vi "Fetch Waveform.vi"(7 "Bind Source Channel (2: None)":i32(ring)=2 items=["Sub Source 0", "Sub Source 1", "None"], 8 "error in (no error)":errorcluster, 9 "Timeout (10000)":u32=10000, 10 "Source Channel (0: Channel 1)":i32(ring) items=["Channel 1"=0, "Channel 2"=1, "Channel 3"=2, "Channel 4"=3, "Waveform Memory 1"=5, "Waveform Memory 2"=6, "Serial Bus 1"=7, "Serial Bus 2"=8, "Digital Bus Low"=9, "Digital Bus High "=10, "Digital Bus 1"=11, "Digital Bus 2"=12, "External"=29, "Function 1"=32, "Function 2"=33, "Function 3"=34, "Function 4"=35, "Math 1"=36, "Math 2"=37, "Math 3"=38, "Math 4"=39, "FFT"=40, "Analog Bus"=41, "Pod 1"=42, "Pod 2"=43], 11 "VISA resource name":refnum<visa-resource-name>) -> (0 "error out":errorcluster, 2 "Waveform Data":waveform(dbl)(graph), 3 "VISA resource name out":refnum<visa-resource-name>)   [LabVIEW 2015, in "Agilent 2000 3000 X-Series.lvlib"]
doc: "Returns the waveform the oscilloscope acquired for the specified channel. The waveform is from an acquisition that you initiate prior to calling this VI.\n\nYou use the <b>Initiate</b> VI to start an acquisition on the channels that you enable with the <b>Configure Channel</b> VI. The oscilloscope acquires waveforms for the enabled channels concurrently. You must call this VI separately for each enabled channel to obtain the waveforms.\n\nYou can call the <b>Read Waveform</b> VI instead of using low-level VIs.\n\n<B>Note(s):</B>\nUse this VI only with other low-level VIs. The high-level VIs automatically incorporate this functionality. This VI does not check the instrument status."
uses:
  Agilent 2000 3000 X-Series.lvlib
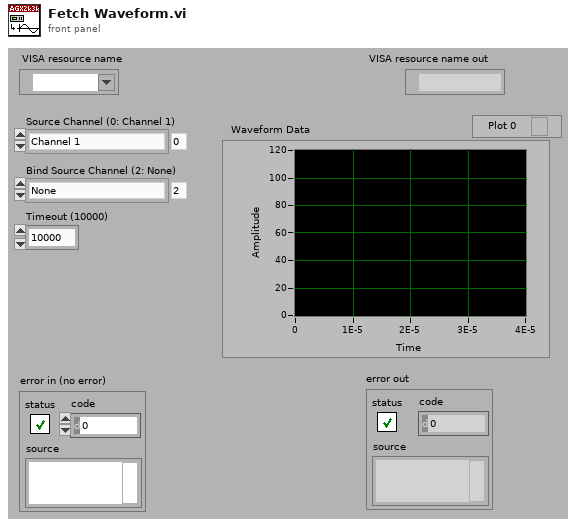
[diagram p1: front panel]
types:
  T1 = typedef "Agilent 2000 3000 X-Series.lvlib/Extended User Data.ctl" = cluster{"X-Series Mode":u16, "Acquisition Type (0: Normal)":i32}
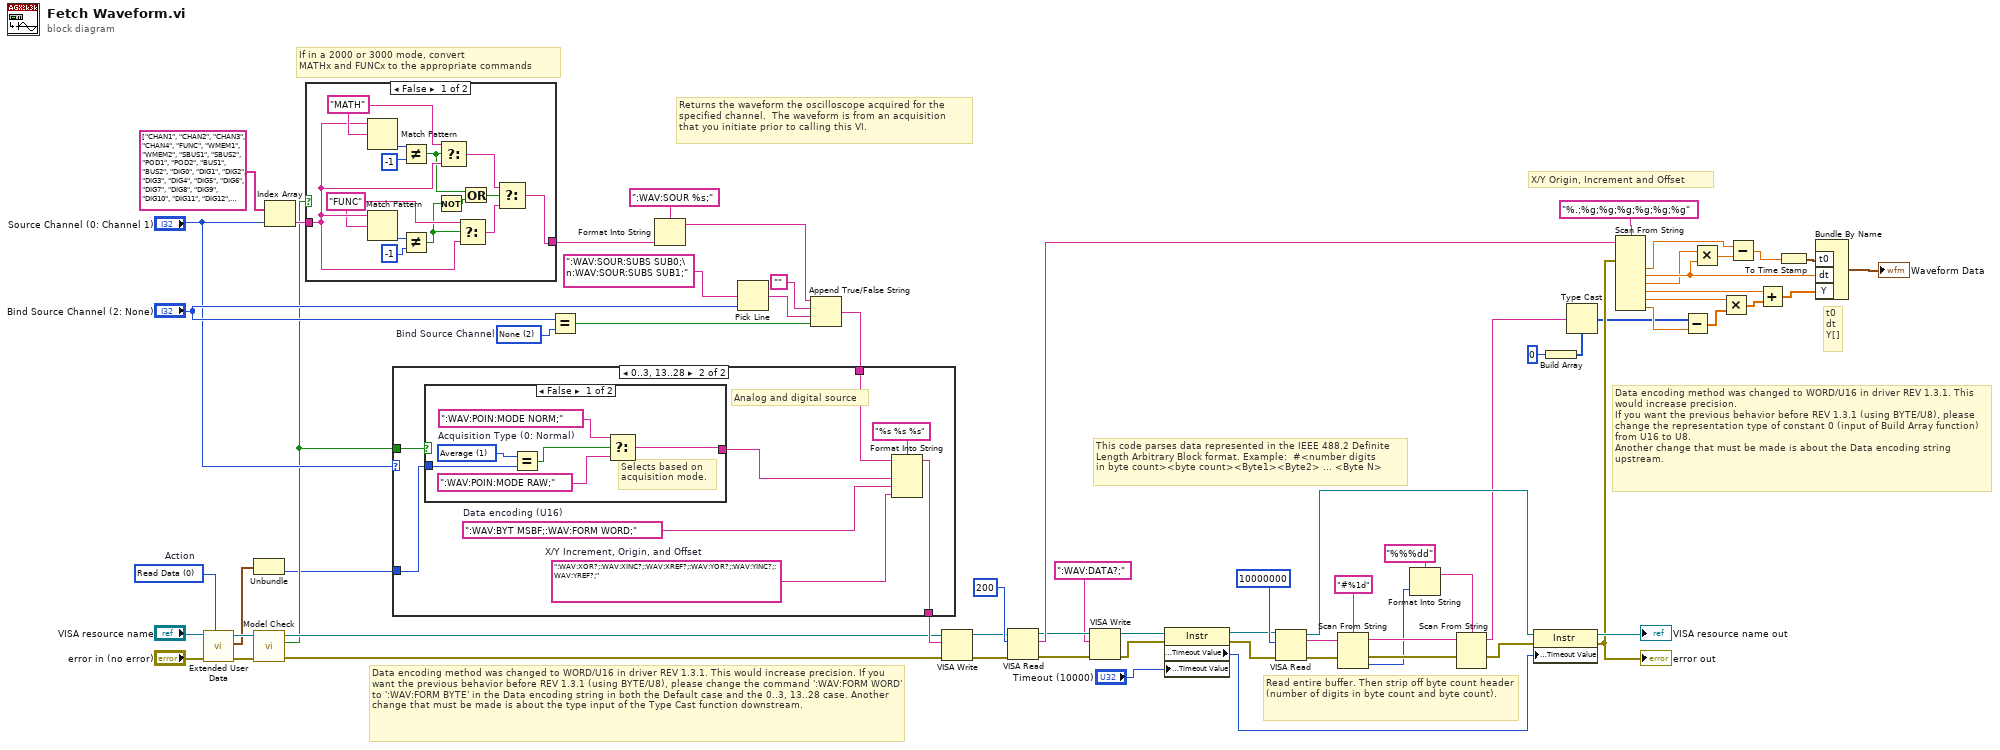
[diagram p0: block diagram]
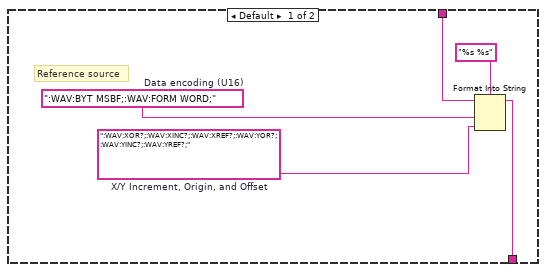
[diagram p3: hidden frame]
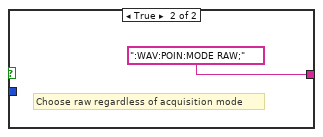
[diagram p4: hidden frame]
diagram:
  w4 = 0 items=["Read Data", "Write Data", "Clear Data", "Clear ALL Data"]  # Action
  w24 = 2 items=["Sub Source 0", "Sub Source 1", "None"]  # Bind Source Channel
  # "Data encoding method was changed to WORD/U16 in driver REV 1.3.1. This would increase precision. If you want the previous behavior before REV 1.3.1 (using BYTE/U8), please change the command ':WAV:FORM WORD' to ':WAV:FORM BYTE' in the Data encoding string in both the Default case and the 0..3, 13..28 case. Another change that must be made is about the type input of the Type Cast function downstream."
  # "Data encoding method was changed to WORD/U16 in driver REV 1.3.1. This would increase precision. \nIf you want the previous behavior before REV 1.3.1 (using BYTE/U8), please change the representation type of constant 0 (input of Build Array function) from U16 to U8. \nAnother change that must be made is about the Data encoding string upstream."
  # "If in a 2000 or 3000 mode, convert\nMATHx and FUNCx to the appropriate commands"
  # "Read entire buffer. Then strip off byte count header (number of digits in byte count and byte count)."
  # "This code parses data represented in the IEEE 488.2 Definite \nLength Arbitrary Block format. Example:  #<number digits \nin byte count><byte count><Byte1><Byte2> ... <Byte N>"
  # "t0\ndt\nY[]"
  # "X/Y Origin, Increment and Offset"
  # "Returns the waveform the oscilloscope acquired for the \nspecified channel.  The waveform is from an acquisition \nthat you initiate prior to calling this VI."
  n1 = call "Extended User Data.vi"("Action (1: Write Data)"=w4, "error in (no error)"="error in (no error)", "VISA resource name in"="VISA resource name") -> ("error out"=w7:errorcluster, "User Data Out"=w3:T1, "VISA resource name out"=w8:refnum<visa-resource-name>)  [unwired: 6 in]
  n2 = Unbundle(w3) -> ("Acquisition Type (0: Normal)"=w1:i32)  [unwired: 1 out]
  n3 = call "Model Check.vi"("error in (no error)"=w7, "VISA resource name"=w8) -> ("error out"=w11:errorcluster, "Not 2000 or 3000 Series"=w2:bool, "VISA resource name out"=w12:refnum<visa-resource-name>)  [unwired: 6 in, 1 out]
  n4 = Index Array(array=string[] ["CHAN1", "CHAN2", "CHAN3", "CHAN4", "FUNC", "WMEM1", "WMEM2", "SBUS1", "SBUS2", "POD1", "POD2", "BUS1", "BUS2", "DIG0", "DIG1", "DIG2", "DIG3", "DIG4", "DIG5", "DIG6", "DIG7", "DIG8", "DIG9", "DIG10", "DIG11", "DIG12", "DIG13", "DIG14", "DIG15", "EXT", "LINE", "WGEN", "FUNC1", "FUNC2", "FUNC3", "FUNC4", "MATH1", "MATH2", "MATH3", "MATH4", "FFT", "ABUS", "POD1", "POD2"], index="Source Channel (0: Channel 1)") -> (element=w10:string)
  n5 = case shown="False" w2 {
    tunnel: w10 -> [w77 w83]
    tunnel: [w73 w83] -> w9
    frame False {
      w76 = "FUNC" ("regular expression")
      w80 = "MATH" ("regular expression")
      n6 = Match Pattern(string=w77, regular expression=w80) -> (offset past match=w82:i32)  [unwired: 1 in, 3 out]
      n7 = Match Pattern(string=w77, regular expression=w76) -> (offset past match=w79:i32)  [unwired: 1 in, 3 out]
      n8 = Not Equal?(x=w82, y=-1) -> (x != y?=w71:bool)
      n9 = Not Equal?(x=w79, y=-1) -> (x != y?=w69:bool)
      n10 = Not(x=w69) -> (.not. x?=w70:bool)
      n11 = Select(t=w80, s=w71, f=w77) -> (s? t:f=w75:string)
      n12 = Select(t=w76, s=w69, f=w77) -> (s? t:f=w74:string)
      n13 = Or(x=w71, y=w70) -> (x .or. y?=w72:bool)
      n14 = Select(t=w75, s=w72, f=w74) -> (s? t:f=w73:string)
    }
    frame True {
    }
  }
  n15 = Equal?(x="Bind Source Channel (2: None)", y=w24) -> (x = y?=w22:bool)
  n16 = Format Into String(format string=":WAV:SOUR %s;", w9) -> (resulting string=w14:string)  [unwired: 2 in, 1 out]
  n17 = Pick Line(multi-line string=":WAV:SOUR:SUBS SUB0;\n:WAV:SOUR:SUBS SUB1;", line index="Bind Source Channel (2: None)") -> (output string=w21:string)  [unwired: 1 out]
  n18 = Append True/False String(1:w22, 2:w21, 3:"", 4:w14) -> (0:w19:string)
  n19 = case shown="0..3, 13..28" "Source Channel (0: Channel 1)" {
    tunnel: [w87 w96] -> w67
    tunnel: w19 -> [w84 w94]
    tunnel: w2 -> [_ w90]
    tunnel: w1 -> [_ w89]
    frame Default {
      w85 = ":WAV:XOR?;:WAV:XINC?;:WAV:XREF?;:WAV:YOR?;:WAV:YINC?;:WAV:YREF?;"  # X/Y Increment, Origin, and Offset
      w86 = ":WAV:BYT MSBF;:WAV:FORM WORD;"  # Data encoding (U16)
      # "Reference source"
      n20 = Format Into String(format string="%s %s", initial string=w84, w86, w85) -> (resulting string=w87:string)  [unwired: 1 in, 1 out]
    }
    frame 0..3, 13..28 {
      w93 = ":WAV:XOR?;:WAV:XINC?;:WAV:XREF?;:WAV:YOR?;:WAV:YINC?;:WAV:YREF?;"  # X/Y Increment, Origin, and Offset
      w95 = ":WAV:BYT MSBF;:WAV:FORM WORD;"  # Data encoding (U16)
      # "Analog and digital source"
      n21 = case shown="False" w90 {
        tunnel: [w100 ":WAV:POIN:MODE RAW;"] -> w92
        tunnel: w89 -> [w99 _]
        frame False {
          w98 = 1 items=["Normal", "Average", "High Resolution", "Peak"]  # Acquisition Type (0: Normal)
          # "Selects based on\nacquisition mode."
          n22 = Equal?(x=w98, y=w99) -> (x = y?=w97:bool)
          n23 = Select(t=":WAV:POIN:MODE NORM;", s=w97, f=":WAV:POIN:MODE RAW;") -> (s? t:f=w100:string)
        }
        frame True {
          # "Choose raw regardless of acquisition mode"
        }
      }
      n24 = Format Into String(format string="%s %s %s", initial string=w94, w92, w95, w93) -> (resulting string=w96:string)  [unwired: 1 in, 1 out]
    }
  }
  n25 = VISA Write(VISA resource name=w12, write buffer=w67, error in (no error)=w11) -> (VISA resource name out=w18:refnum<visa-resource-name>, error out=w17:errorcluster)  [unwired: 1 out]
  n26 = VISA Read(VISA resource name=w18, byte count=u32 200, error in (no error)=w17) -> (VISA resource name out=w45:refnum<visa-resource-name>, read buffer=w64:string, error out=w44:errorcluster)  [unwired: 1 out]
  n27 = VISA Write(VISA resource name=w45, write buffer=":WAV:DATA?;", error in (no error)=w44) -> (VISA resource name out=w46:refnum<visa-resource-name>, error out=w47:errorcluster)  [unwired: 1 out]
  n28 = property class="Instr"(reference=w46, error in=w47, "General Settings:Timeout Value"="Timeout (10000)") -> (reference out=w41:refnum<visa-resource-name>, error out=w40:errorcluster, "General Settings:Timeout Value"=w43:u32)
  n29 = VISA Read(VISA resource name=w41, byte count=u32 10000000, error in (no error)=w40) -> (VISA resource name out=w39:refnum<visa-resource-name>, read buffer=w50:string, error out=w48:errorcluster)  [unwired: 1 out]
  n30 = Scan From String(format string="#%1d", input string=w50, error in=w48) -> (remaining string=w54:string, error out=w52:errorcluster, output 1=w51:i32)  [unwired: 1 in, 2 out]
  n31 = Format Into String(format string="%%%dd", w51) -> (resulting string=w53:string)  [unwired: 2 in, 1 out]
  n32 = Scan From String(format string=w53, input string=w54, error in=w52) -> (remaining string=w35:string, error out=w34:errorcluster)  [unwired: 1 in, 3 out]
  n33 = property class="Instr"(reference=w39, error in=w34, "General Settings:Timeout Value"=w43) -> (reference out=→"VISA resource name out":refnum<visa-resource-name>, error out=w33:errorcluster)
  "error out" <- w33
  n34 = Build Array(u16 0) -> (w37:u16[])
  n35 = Type Cast(type=w37, x=w35) -> (*(type *) &x=w30:u16[])
  n36 = Scan From String(format string="%.;%g;%g;%g;%g;%g;%g", input string=w64, error in=w33) -> (output 1=w57:dbl, output 2=w61:dbl, output 3=w60:dbl, output 4=w27:dbl, output 5=w29:dbl, output 6=w31:dbl)  [unwired: 1 in, 9 out]
  n37 = Subtract(x=w30, y=w31) -> (x-y=w28:dbl[])
  n38 = Multiply(x=w60, y=w61) -> (x*y=w58:dbl)
  n39 = Multiply(x=w29, y=w28) -> (x*y=w26:dbl[])
  n40 = Subtract(x=w57, y=w58) -> (x-y=w59:dbl)
  n41 = Add(x=w27, y=w26) -> (x+y=w25:dbl[])
  n42 = To Time Stamp(1:w59) -> (0:w63:timestamp)
  n43 = Bundle By Name("t0"=w63, "dt"=w61, "Y"=w25) -> (→"Waveform Data":waveform(dbl))  [unwired: 1 out]
